vi "Configure Mediator.vi"(9 "Framework Instance Alias":string, 10 "Event Log Instance":refnum<class "LoggerReference.lvclass">, 11 "Mediator in":refnum<class "IMediator.lvclass">) -> (3 "Mediator out":refnum<class "IMediator.lvclass">)   [LabVIEW 2020, in "MVA Framework.lvlib" / "IMediator.lvlib" / "IMediator.lvclass"]
doc: "配置中介"
uses:
  IMediator.lvclass
  composed-event-logger/Source/Composed Log/LoggerReference/LoggerReference.lvclass
  IMediator.lvclass/IMediator.ctl
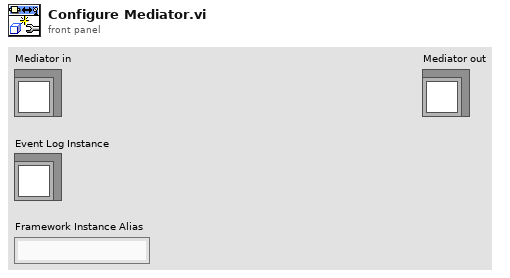
[diagram p1: front panel]
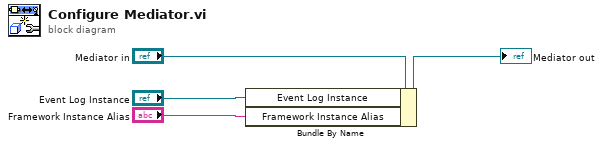
[diagram p0: block diagram]
diagram:
  n1 = Bundle By Name(cluster="Mediator in", "Event Log Instance"="Event Log Instance", "Framework Instance Alias"="Framework Instance Alias") -> (→"Mediator out":refnum<class "IMediator.lvclass">)
